vi "Black_box.vi"() -> (0 "error out":errorcluster, 3 "task out":refnum<k21>)   [LabVIEW 2014]
uses:
  <vilib>/DAQmx/create/channels.llb/DAQmx Create Channel (AI-Voltage-Basic).vi
  <vilib>/DAQmx/configure/timing.llb/DAQmx Timing (Sample Clock).vi
panel:
  in  "Sampling Rate":dbl=1000.0 format="%0.2f"
  in  "auto cleanup":bool
  in  "error in":errorcluster
  in  "KEEP THIS TURNED ON":bool
  in  "Samples / Channel":i32=1000
  in  "Sampling Mode":i32(ring)=10178 items=["Finite Samples"=10178, "Continuous Samples"=10123, "Hardware Timed Single Point"=12522]
  in  "Encoder":tag
  in  "min V":dbl=-5.0 format="%0.2f"
  in  "max V":dbl=5.0 format="%0.2f"
  in  "max V":dbl=5.0 format="%0.2f"
  in  "min V":dbl=-5.0 format="%0.2f"
  in  "LVDT1":tag
  in  "max V":dbl=5.0 format="%0.2f"
  in  "min V":dbl=-5.0 format="%0.2f"
  in  "LVDT2":tag
  in  "Bottom Load Celll":tag
  in  "min V":dbl=-5.0 format="%0.2f"
  in  "max V":dbl=5.0 format="%0.2f"
  in  "Top Load Cell":tag
  in  "min V":dbl=-5.0 format="%0.2f"
  in  "max V":dbl=5.0 format="%0.2f"
  in  "max V":dbl=5.0 format="%0.2f"
  in  "min V":dbl=-5.0 format="%0.2f"
  in  "Torqe Transducer":tag
  in  "min V":dbl=-5.0 format="%0.2f"
  in  "max V":dbl=5.0 format="%0.2f"
  in  "Monitor Input":tag
  # "The Black Box\n\n7 channels  and set up as an I/O \n\n [as a Sub-Vi]"
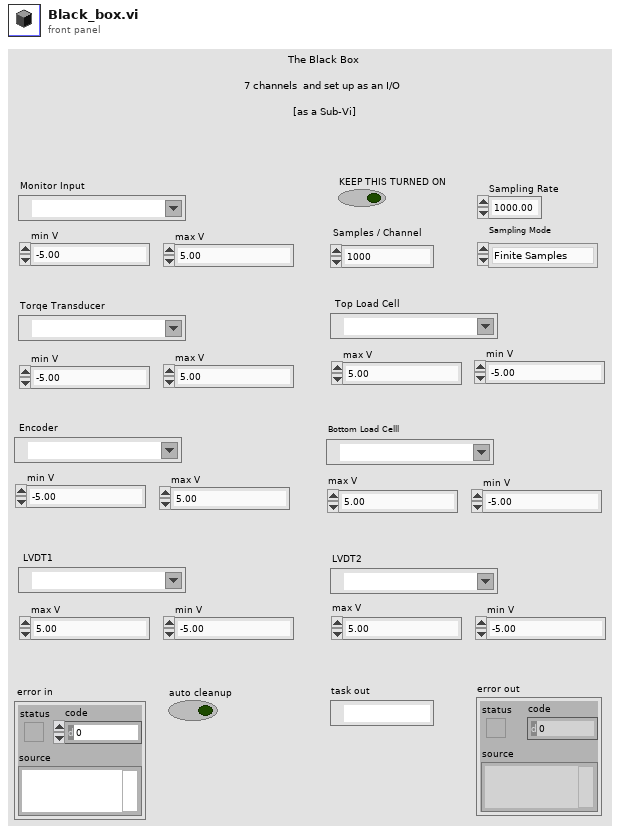
[diagram p1: front panel]
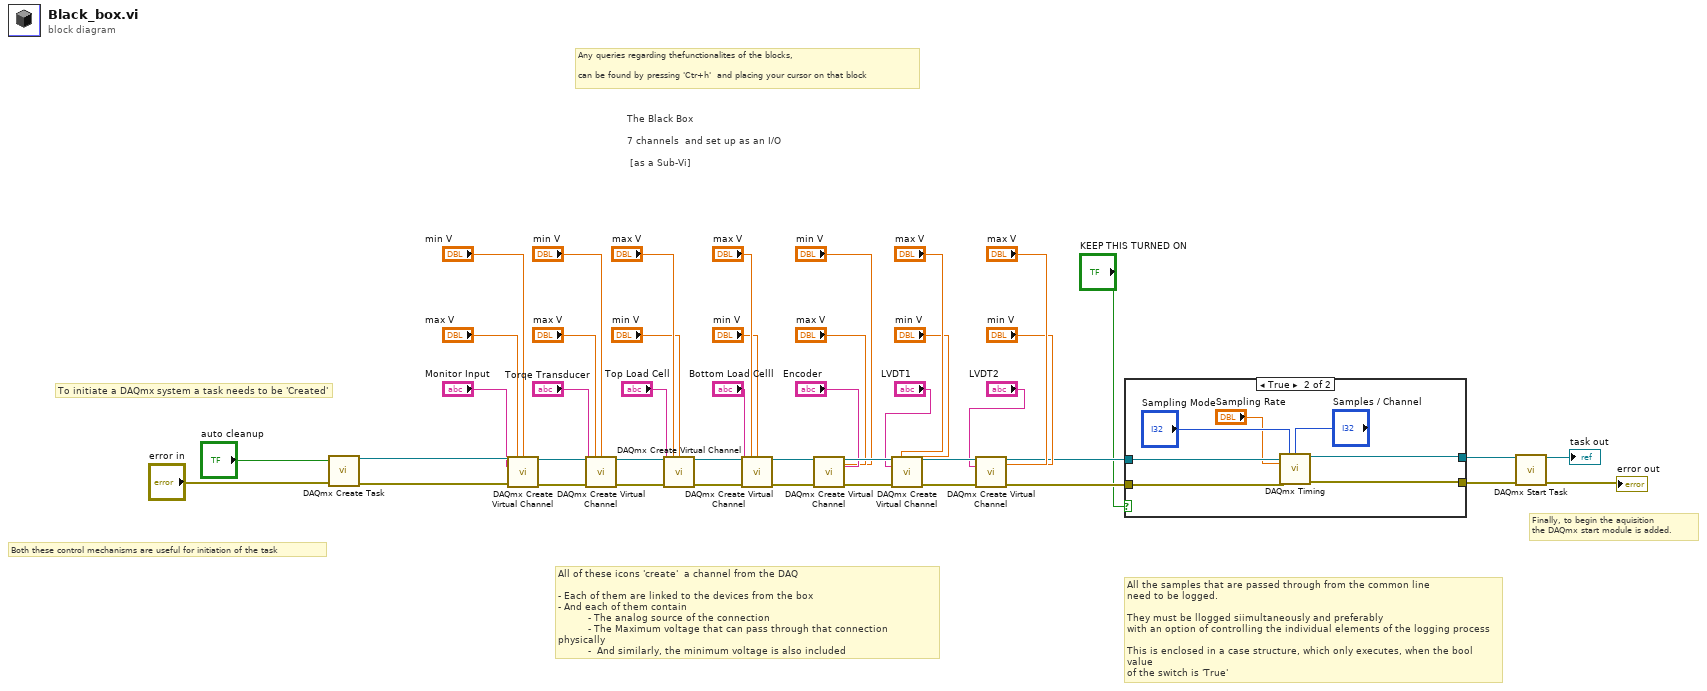
[diagram p0: block diagram]
diagram:
  # "Any queries regarding thefunctionalites of the blocks, \n\ncan be found by pressing 'Ctr+h'  and placing your cursor on that block"
  # "Finally, to begin the aquisition\nthe DAQmx start module is added."
  # "All the samples that are passed through from the common line\nneed to be logged.\n\nThey must be llogged siimultaneously and preferably \nwith an option of controlling the individual elements of the logging process\n\nThis is enclosed in a case structure, which only executes, when the bool value\nof the switch is 'True'"
  # "All of these icons 'create'  a channel from the DAQ\n\n- Each of them are linked to the devices from the box\n- And each of them contain \n          - The analog source of the connection\n          - The Maximum voltage that can pass through that connection physically \n          -  And similarly, the minimum voltage is also included"
  # "Both these control mechanisms are useful for initiation of the task"
  # "To initiate a DAQmx system a task needs to be 'Created'"
  # "The Black Box\n\n7 channels  and set up as an I/O \n\n [as a Sub-Vi]"
  n1 = call <vilib>:"DAQmx Create Task.vi"("auto cleanup"="auto cleanup", "error in"="error in") -> ("task out"=w37:refnum<k21>, "error out"=w44:errorcluster)  [unwired: 12 in]
  n2 = call-poly <vilib>:"DAQmx Create Virtual Channel.vi"("task in"=w37, "maximum value"="max V", "minimum value"="min V", "physical channels"="Monitor Input", "error in"=w44) -> ("task out"=w36:refnum<k21>, "error out"=w43:errorcluster)  [unwired: 9 in]
  n3 = call-poly <vilib>:"DAQmx Create Virtual Channel.vi"("task in"=w36, "maximum value"="max V", "minimum value"="min V", "physical channels"="Torqe Transducer", "error in"=w43) -> ("task out"=w35:refnum<k21>, "error out"=w42:errorcluster)  [unwired: 9 in]
  n4 = call-poly <vilib>:"DAQmx Create Virtual Channel.vi"("task in"=w35, "maximum value"="max V", "minimum value"="min V", "physical channels"="Top Load Cell", "error in"=w42) -> ("task out"=w34:refnum<k21>, "error out"=w41:errorcluster)  [unwired: 9 in]
  n5 = call-poly <vilib>:"DAQmx Create Virtual Channel.vi"("task in"=w34, "maximum value"="max V", "minimum value"="min V", "physical channels"="Bottom Load Celll", "error in"=w41) -> ("task out"=w33:refnum<k21>, "error out"=w40:errorcluster)  [unwired: 9 in]
  n6 = call-poly <vilib>:"DAQmx Create Virtual Channel.vi"("task in"=w33, "maximum value"="max V", "minimum value"="min V", "physical channels"="Encoder", "error in"=w40) -> ("task out"=w32:refnum<k21>, "error out"=w39:errorcluster)  [unwired: 9 in]
  n7 = call-poly <vilib>:"DAQmx Create Virtual Channel.vi"("task in"=w32, "maximum value"="max V", "minimum value"="min V", "physical channels"="LVDT1", "error in"=w39) -> ("task out"=w31:refnum<k21>, "error out"=w38:errorcluster)  [unwired: 9 in]
  n8 = call-poly <vilib>:"DAQmx Create Virtual Channel.vi"("task in"=w31, "maximum value"="max V", "minimum value"="min V", "physical channels"="LVDT2", "error in"=w38) -> ("task out"=w9:refnum<k21>, "error out"=w8:errorcluster)  [unwired: 9 in]
  n9 = case shown="True" "KEEP THIS TURNED ON" {
    tunnel: w9 -> [w46 w53]
    tunnel: w8 -> [w45 w51]
    tunnel: [w46 w52] -> w6
    tunnel: [w45 w50] -> w5
    frame False {
    }
    frame True {
      n10 = call-poly <vilib>:"DAQmx Timing.vi"("task/channels in"=w53, "sample mode"="Sampling Mode", "samples per channel"="Samples / Channel", "rate"="Sampling Rate", "error in"=w51) -> ("task out"=w52:refnum<k21>, "error out"=w50:errorcluster)  [unwired: 9 in]
    }
  }
  n11 = call <vilib>:"DAQmx Start Task.vi"("task/channels in"=w6, "error in"=w5) -> ("task out"=→"task out":refnum<k21>, "error out"=→"error out":errorcluster)  [unwired: 12 in]
